vi "Lookup Channel.vi"(7 "VolatusAPI":refnum<class "VolatusAPI.lvclass">, 8 "error in (no error)":errorcluster, 9 "Name":string, 11 "Channels in":map{string, T1}(c390)) -> (0 "error out":errorcluster, 1 "Value":dbl, 2 "Redline":bool, 3 "Channels":map{string, T1}(c390))   [LabVIEW 2020, in "VolatusGUIElements.lvlib" / "BluelinesRedlines.lvclass"]
uses:
  BluelinesRedlines.lvclass
  lv-vecto/Vecto/Channel DBL/Channel DBL.lvclass
  Volatus/VolatusAPI/VolatusAPI.lvclass
  Volatus/VolatusAPI/VolatusAPI.lvclass/VolatusAPI.ctl
  lv-vecto/Vecto/Channel DBL/Channel DBL.lvclass/Channel DBL.ctl
  lv-vecto/Vecto/ChannelService/Lookup Double Channel.vi
  lv-vecto/Vecto/Group DBL/Value by Index.vi
  BluelinesRedlines.lvclass/BluelinesRedlines.ctl
  Channel Info.ctl
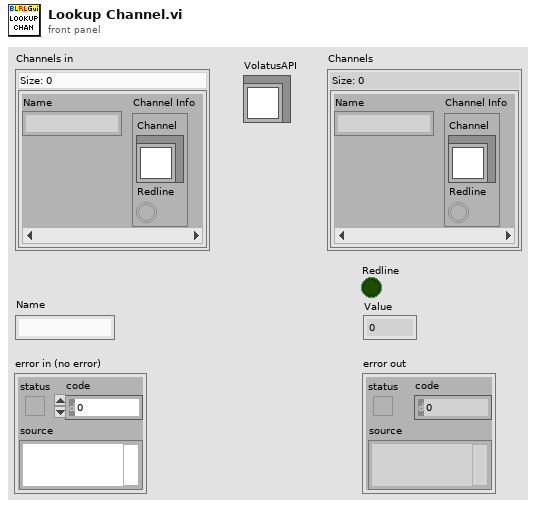
[diagram p1: front panel]
types:
  T1 = typedef "VolatusGUIElements.lvlib/BluelinesRedlines.lvclass/Channel Info.ctl" = cluster{"Channel":refnum<class "Channel DBL.lvclass">, "Redline":bool}
  T2 = cluster{"Channel DBL":refnum<class "Channel DBL.lvclass">, bool}
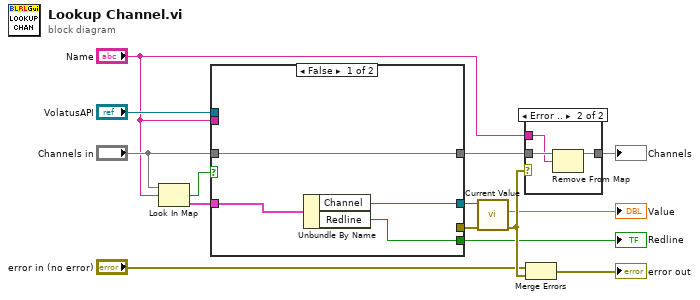
[diagram p0: block diagram]
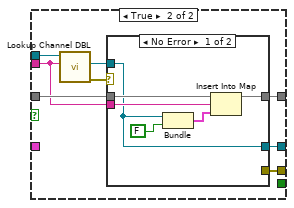
[diagram p3: hidden frame]
diagram:
  n1 = Look In Map(map="Channels in", key="Name") -> (key not found?=w12:bool, value=w11:T1)  [unwired: 1 in]
  n2 = case shown="False" w12 {
    tunnel: w11 -> [w18 _]
    tunnel: "Channels in" -> [w17 w23]
    tunnel: "Name" -> [_ w22]
    tunnel: "VolatusAPI" -> [_ w26]
    tunnel: [w17 w21] -> w4
    tunnel: [w16 w19] -> w8
    tunnel: [_ w20] -> w6
    tunnel: [w15 _] -> w1
    frame False {
      n3 = Unbundle By Name(w18) -> ("Channel"=w16:refnum<class "Channel DBL.lvclass">, "Redline"=w15:bool)
    }
    frame True {
      n4 = call "Lookup Channel DBL.vi"("Name"=w22, "VolatusAPI in"=w26) -> ("error out"=w25:errorcluster, "Channel DBL"=w24:refnum<class "Channel DBL.lvclass">)  [unwired: 7 in, 1 out]
      n5 = case shown="No Error" w25 {
        selector: w25 -> [_ w34]
        tunnel: w24 -> [w29 _]
        tunnel: w23 -> [w32 w33]
        tunnel: w22 -> [w31 _]
        tunnel: [w30 w33] -> w21
        tunnel: [_ w34] -> w20
        tunnel: [w29 _] -> w19
        frame No Error {
          n6 = Bundle("Channel DBL"=w29, FALSE) -> (w27:T2)  [unwired: 1 in]
          n7 = Insert Into Map(map in=w32, key=w31, value=w27) -> (map out=w30:map{string, T1})  [unwired: 2 out]
        }
        frame Error {
        }
      }
    }
  }
  "Redline" <- w1
  n8 = call "Current Value.vi"("error in (no error)"=w6, "Channel in"=w8) -> ("error out"=w14:errorcluster, "Scaled"=→"Value":dbl)  [unwired: 5 in, 3 out]
  n9 = case shown="Error .." w14 {
    tunnel: w4 -> [w35 w38]
    tunnel: "Name" -> [_ w37]
    tunnel: [w35 w36] -> w2
    frame No Error {
    }
    frame Error {
      n10 = Remove From Map(10:w37, 11:w38) -> (3:w36:map{string, T1})  [unwired: 2 out]
    }
  }
  "Channels" <- w2
  n11 = Merge Errors("error in (no error)", w14) -> (→"error out":errorcluster)
